vi "HOST Sample.vi"() -> ()   [LabVIEW 2014]
uses:
  <resource>/objmgr/ni.dex.rc
panel:
  out "Is Connected":bool
  out "error out 2":errorcluster
  out "Stop":bool
  out "Waveform Chart":dbl[](graph)
  out "error out":errorcluster
  in  "Data":string
  in  "Send":bool
  in  "Stop":bool
  in  "Connect":bool
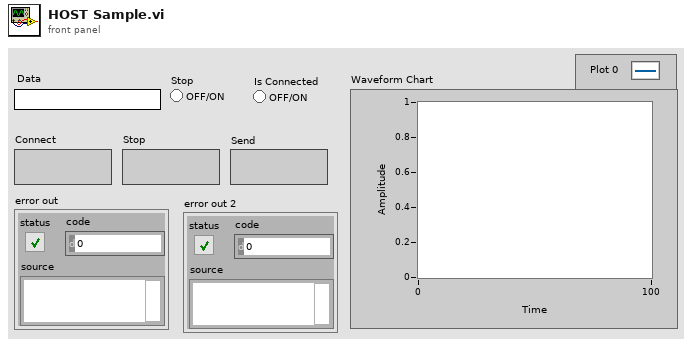
[diagram p1: front panel]
types:
  T1 = enum8{"Enabled", "Disabled", "Disabled and Grayed Out"}
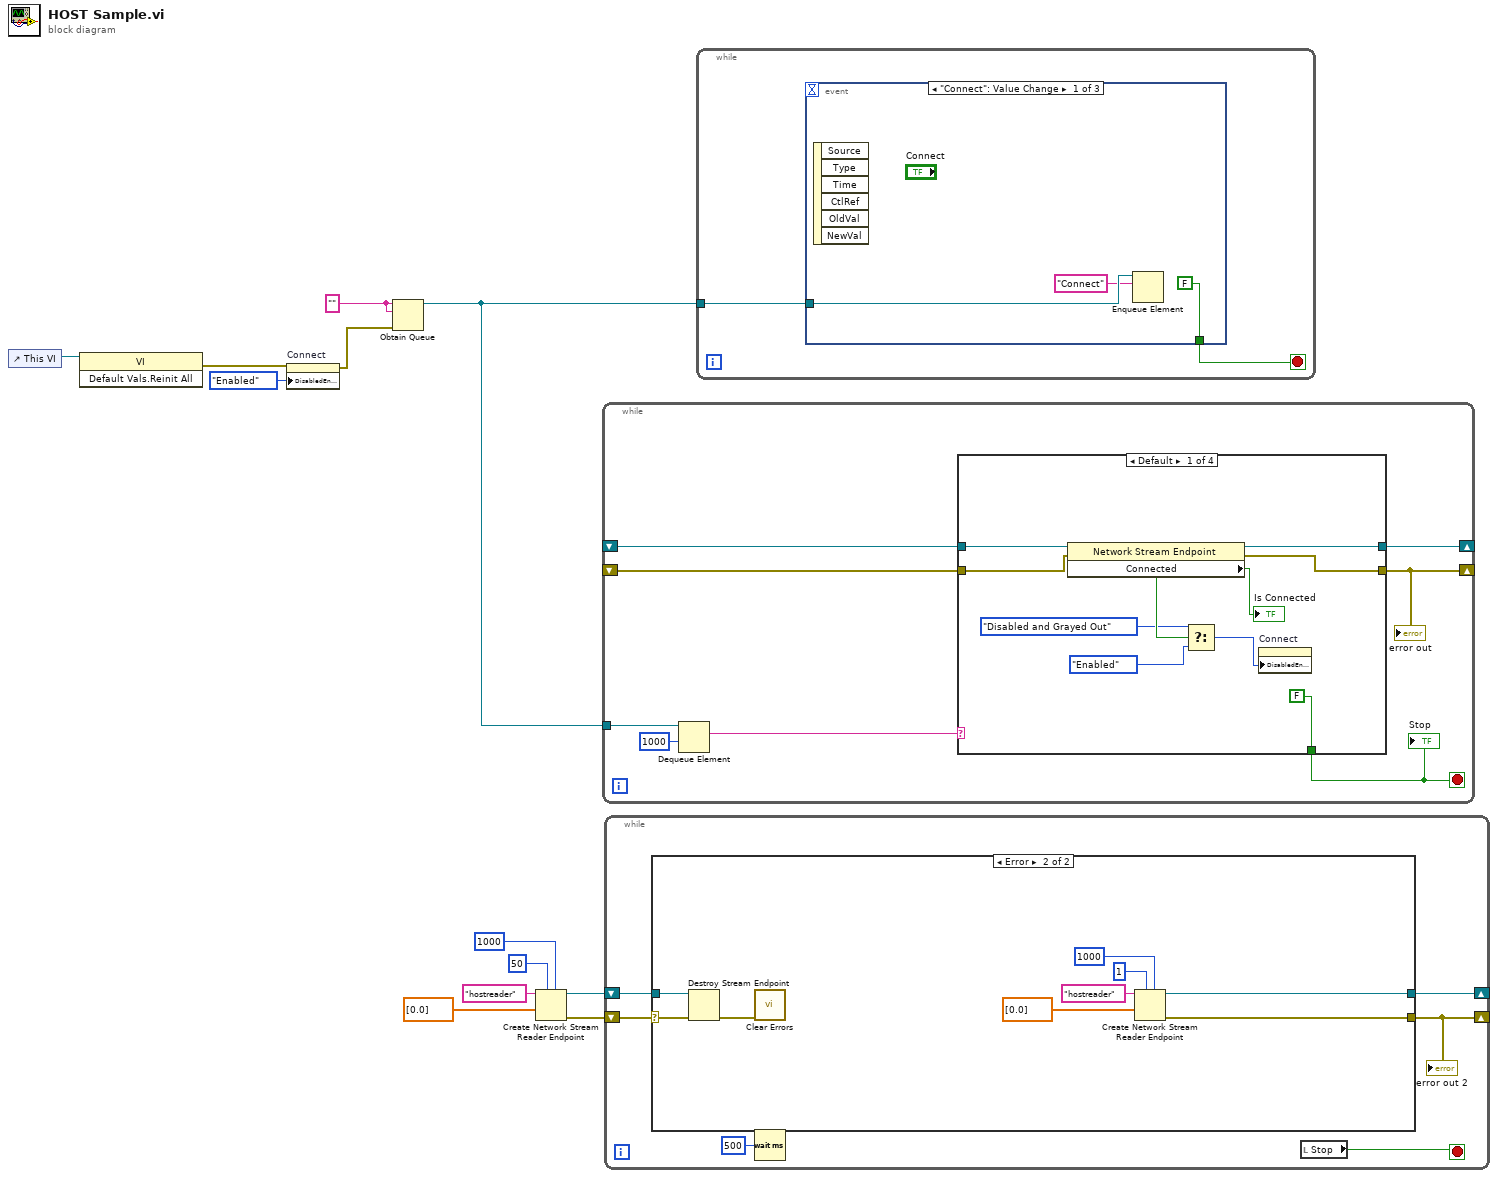
[diagram p0: block diagram]
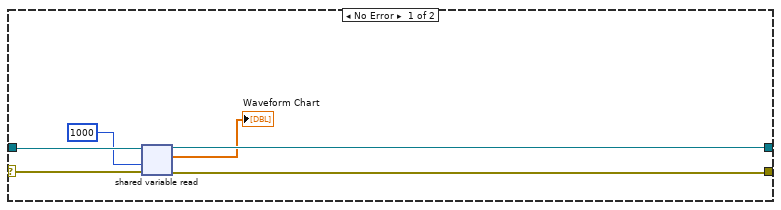
[diagram p2: hidden frame]
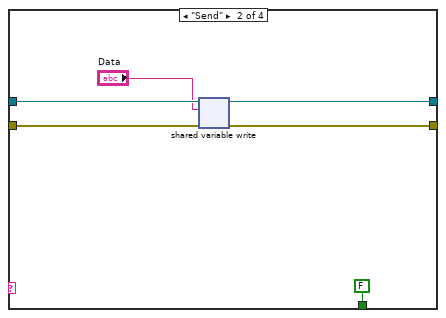
[diagram p3: hidden frame]
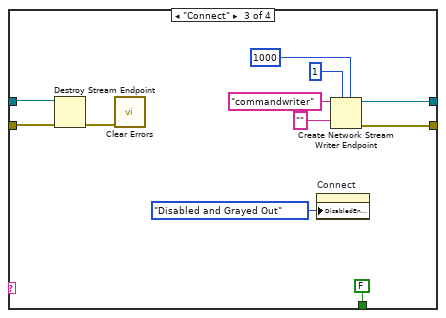
[diagram p4: hidden frame]
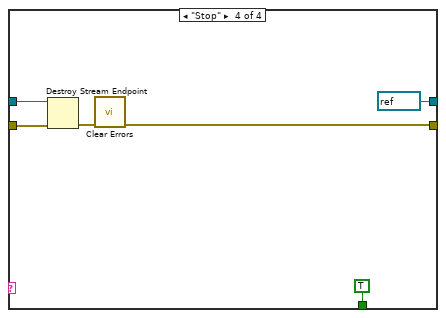
[diagram p5: hidden frame]
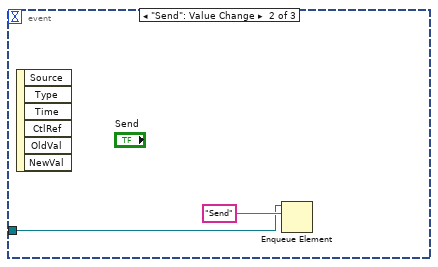
[diagram p6: hidden frame]
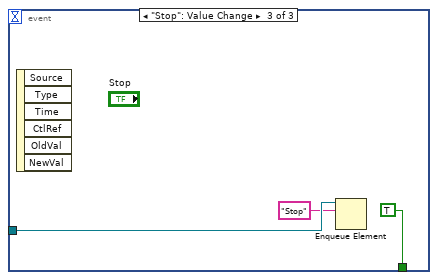
[diagram p7: hidden frame]
diagram:
  w11 = ""
  n1 = control-ref of="This VI"() -> (w2:refnum<vi>)
  n2 = invoke class="VI" method="Default Vals.Reinit All"(reference=w2) -> (error out=w1:errorcluster)  [unwired: 2 in, 2 out]
  n3 = property on="Connect" class="Bool"(error in=w1, "DisabledEnum"=T1."Enabled" ("Disabled")) -> (error out=w9:errorcluster)  [unwired: 1 in, 1 out]
  n4 = Obtain Queue(name (unnamed)=w11, element data type=w11, error in (no error)=w9) -> (queue out=w12:refnum<queue>)  [unwired: 2 in, 2 out]
  n5 = Create Network Stream Reader Endpoint(5:1000 ("timeout in ms (-1)"), 7:50 ("reader buffer size"), 9:dbl[] [0.0], 11:"hostreader" ("reader name")) -> (0:w4:errorcluster, 3:w5:refnum<k21>)  [unwired: 3 in]
  n6 = while {
    tunnel: w12 -> [w20]
    shift-right: [w17] -> _
    shift-left: _ -> [w14]
    shift-right: [w16] -> _
    shift-left: _ -> [w13]
    stop <- w18 stop-if-true
    n7 = Dequeue Element(queue=w20, timeout in ms (-1)=1000) -> (element=w19:string)  [unwired: 1 in, 3 out]
    n8 = case shown="Default" w19 {
      tunnel: [FALSE FALSE FALSE TRUE] -> w18
      tunnel: [w27 w35 w42 refnum<k21> refnum ("writer name")] -> w17
      tunnel: [w25 w32 w40 w49] -> w16
      tunnel: w14 -> [w28 w34 w38 w48]
      tunnel: w13 -> [w26 w33 w37 w50]
      frame Default {
        n9 = property class="Network Stream Endpoint"(reference=w28, error in=w26) -> (reference out=w27:refnum<k21>, error out=w25:errorcluster, "Connected"=w24:bool)
        "Is Connected" <- w24
        n10 = Select(t=T1."Disabled and Grayed Out" ("Disabled"), s=w24, f=T1."Enabled" ("Disabled")) -> (s? t:f=w21:T1)
        n11 = property on="Connect" class="Bool"("DisabledEnum"=w21) -> ()  [unwired: 2 in, 2 out]
      }
      frame "Send" {
        n12 = shared-variable-write(w34, w33, "Data") -> (w35:refnum<k21>, w32:errorcluster)  [unwired: 1 in, 1 out]
      }
      frame "Connect" {
        n13 = Destroy Stream Endpoint(8:w37, 11:w38) -> (0:w36:errorcluster)
        n14 = call <vilib>:"Clear Errors.vi"("error in (no error)"=w36) -> ()  [unwired: 5 in, 2 out]
        n15 = property on="Connect" class="Bool"("DisabledEnum"=T1."Disabled and Grayed Out" ("Disabled")) -> ()  [unwired: 2 in, 2 out]
        n16 = Create Network Stream Writer Endpoint(5:1000 ("timeout in ms (-1)"), 7:1 ("writer buffer size"), 9:"" ("writer name"), 11:"commandwriter" ("writer name")) -> (0:w40:errorcluster, 3:w42:refnum<k21>)  [unwired: 3 in]
      }
      frame "Stop" {
        n17 = Destroy Stream Endpoint(8:w50, 11:w48) -> (0:w51:errorcluster)
        n18 = call <vilib>:"Clear Errors.vi"("error in (no error)"=w51) -> ("error out"=w49:errorcluster)  [unwired: 5 in, 1 out]
      }
    }
    "error out" <- w16
    "Stop" <- w18
  }
  n19 = while {
    shift-right: [w56] -> _
    shift-left: w5 -> [w57]
    shift-right: [w55] -> _
    shift-left: w4 -> [w58]
    stop <- w54 stop-if-true
    n20 = case shown="Error" w58 {
      selector: w58 -> [w63 w73]
      tunnel: w57 -> [w64 w72]
      tunnel: [w62 w66] -> w56
      tunnel: [w61 w65] -> w55
      frame No Error {
        n21 = shared-variable-read(w64, w63, 1000 ("timeout ms (-1)")) -> (w62:refnum<k21>, w61:errorcluster, →"Waveform Chart":dbl[])  [unwired: 1 out]
      }
      frame Error {
        n22 = Destroy Stream Endpoint(8:w73, 11:w72) -> (0:w71:errorcluster)
        n23 = call <vilib>:"Clear Errors.vi"("error in (no error)"=w71) -> ()  [unwired: 5 in, 2 out]
        n24 = Create Network Stream Reader Endpoint(5:1000 ("timeout in ms (-1)"), 7:1 ("reader buffer size"), 9:dbl[] [0.0], 11:"hostreader" ("reader name")) -> (0:w65:errorcluster, 3:w66:refnum<k21>)  [unwired: 3 in]
      }
    }
    "error out 2" <- w55
    n25 = Wait (ms)(milliseconds to wait=u32 500) -> ()  [unwired: 1 out]
    n26 = local read "Stop"() -> (w54:bool)
  }
  n27 = while {
    tunnel: w12 -> [w75]
    stop <- w74 stop-if-true
    n28 = event shown="[0] \"Connect\": Value Change" {
      selector: _ -> [_ _ _]
      dyn-events: _ -> [_ _ _]
      timeout: _ -> [_ _ _]
      tunnel: w75 -> [w78 w79 w83]
      tunnel: [FALSE _ TRUE] -> w74
      event "Connect": Value Change {
        n29 = event-data() -> ()  [unwired: 1 in, 6 out]
        n30 = Enqueue Element(queue=w78, element="Connect") -> ()  [unwired: 2 in, 3 out]
      }
      event "Send": Value Change {
        n31 = event-data() -> ()  [unwired: 1 in, 6 out]
        n32 = Enqueue Element(queue=w79, element="Send") -> ()  [unwired: 2 in, 3 out]
      }
      event "Stop": Value Change {
        n33 = event-data() -> ()  [unwired: 1 in, 6 out]
        n34 = Enqueue Element(queue=w83, element="Stop") -> ()  [unwired: 2 in, 3 out]
      }
    }
  }
